vi "Project 11 - MHJ.vi"() -> ()   [LabVIEW 2019]
uses:
  Control 1.ctl
  <vilib>/Waveform/WDTOps.llb/WDT Number of Waveform Samples DBL.vi
  <vilib>/Waveform/WDTOps.llb/WDT Get Waveform Subset DBL.vi
panel:
  out "# Keypad":T1
  in  "Mode":bool
  out "Waveform Chart":dynamicdata(graph)
  in  "stop":bool
  in  "Waveform":waveform(dbl)
  in  "Load File":bool
  out "String":string
  out "Collected Signals":dynamicdata(graph)
  # "RAW SIGNAL"
  # "COLLECTED SIGNAL"
  # "LOAD"
  # "RAW"
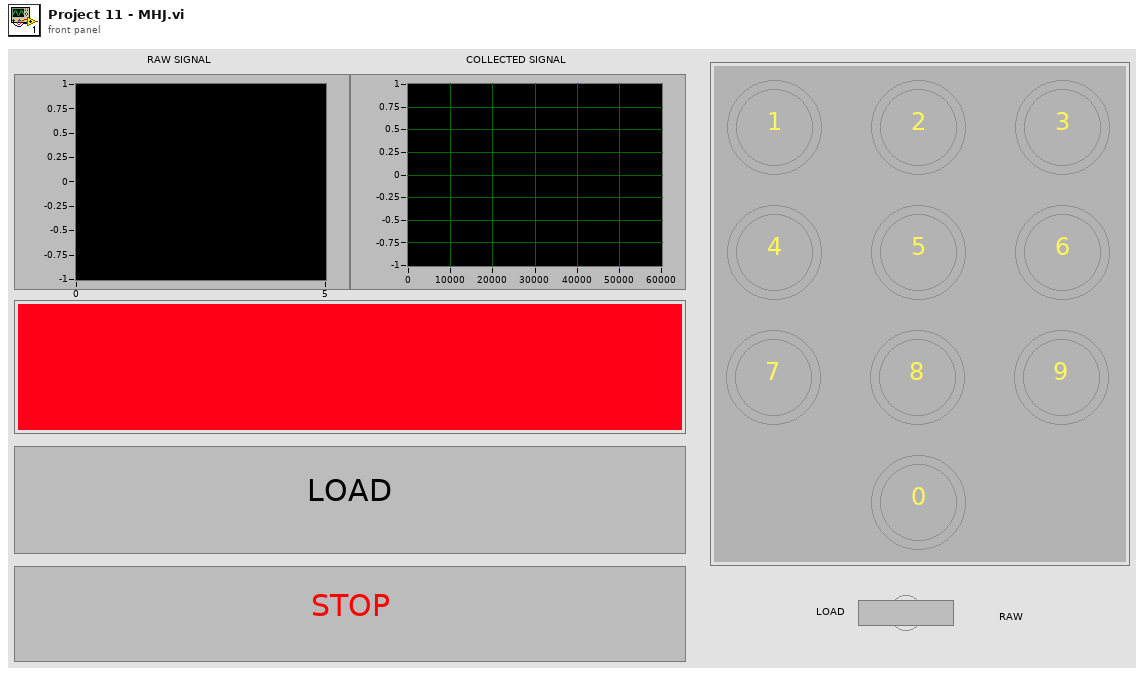
[diagram p1: front panel]
types:
  T1 = cluster{"Boolean 0":bool, "Boolean 9":bool, "Boolean 8":bool, "Boolean 7":bool, "Boolean 6":bool, "Boolean 5":bool, "Boolean 4":bool, "Boolean 3":bool, "Boolean 2":bool, "Boolean 1":bool}
  T2 = typedef "Control 1.ctl" = enum16{"Idle", "Load Image", "Process"}
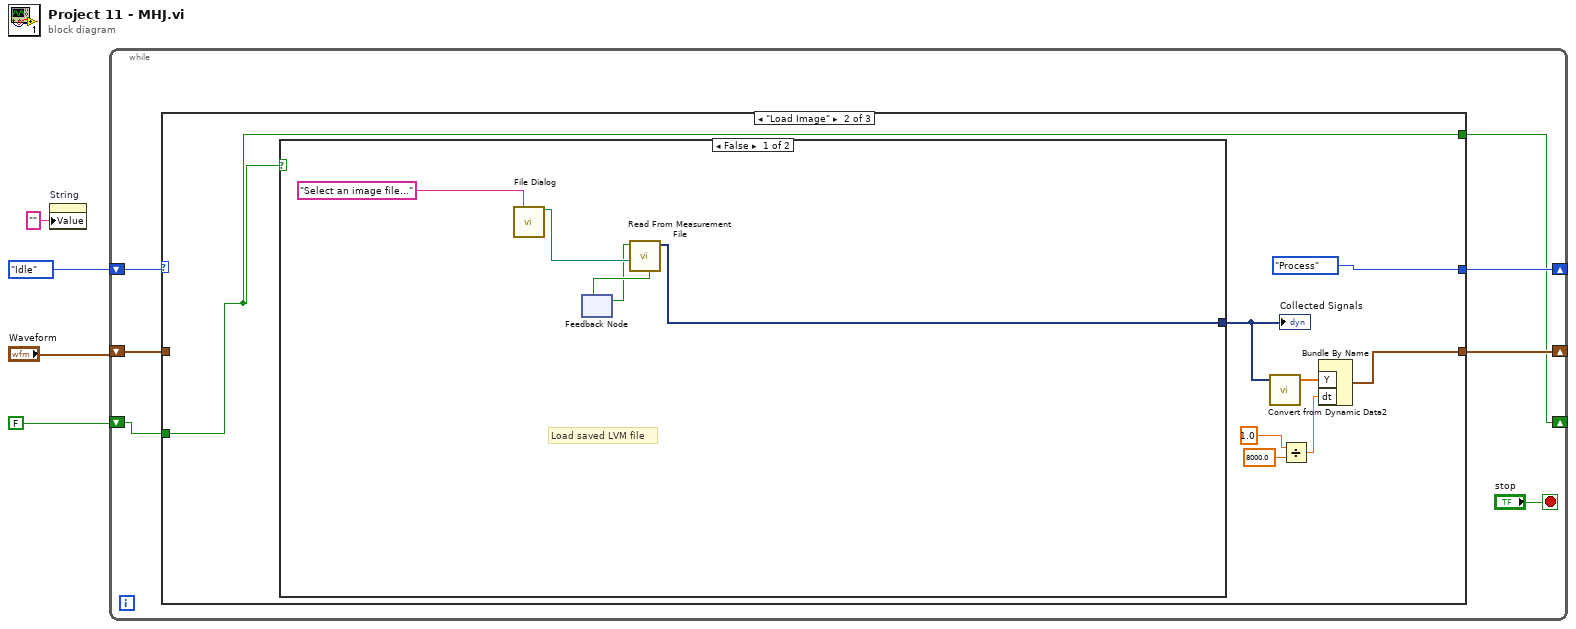
[diagram p0: block diagram]
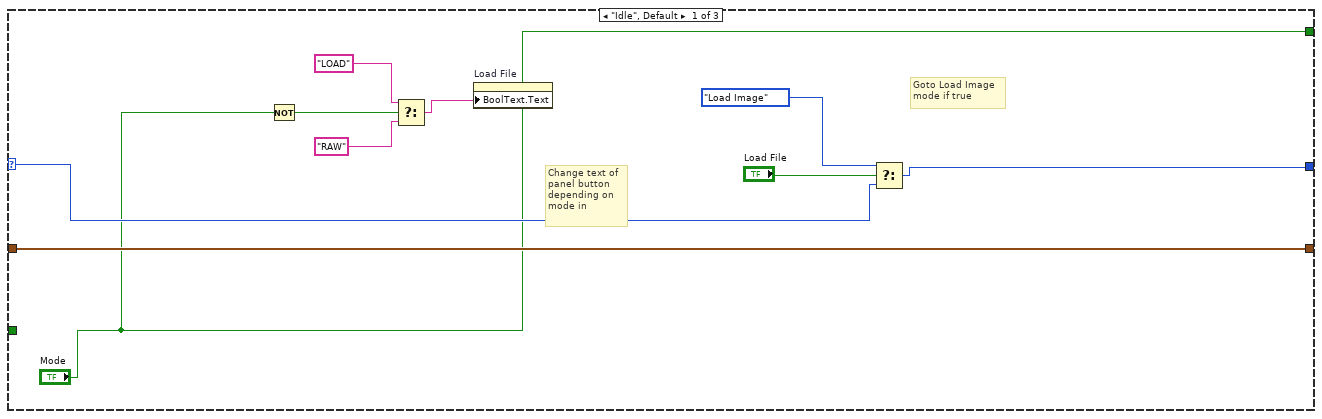
[diagram p2: hidden frame]
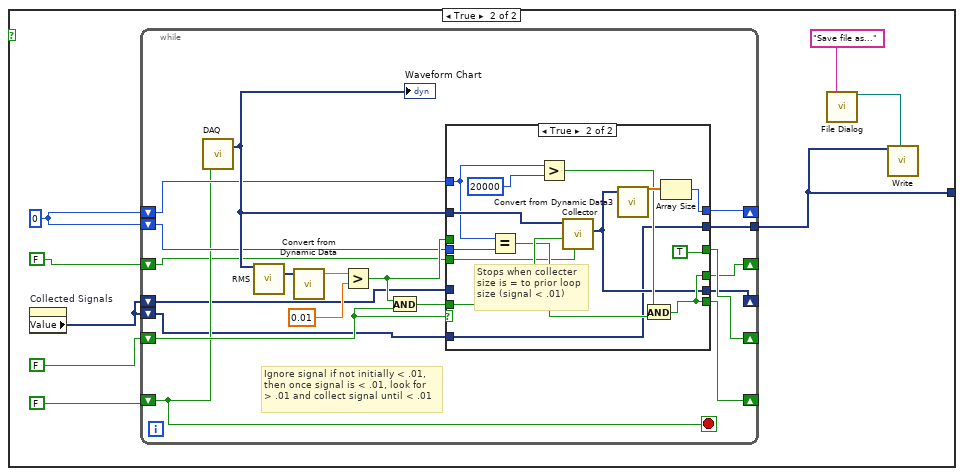
[diagram p3: hidden frame]
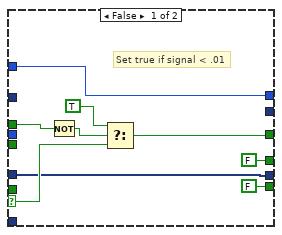
[diagram p4: hidden frame]
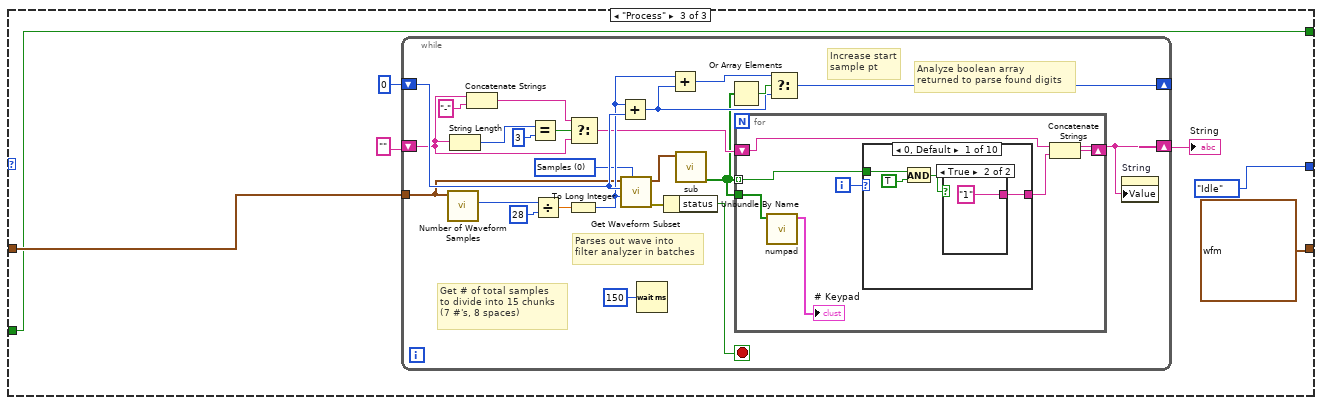
[diagram p5: hidden frame]
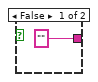
[diagram p6: hidden frame]
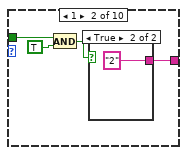
[diagram p7: hidden frame]
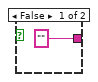
[diagram p8: hidden frame]
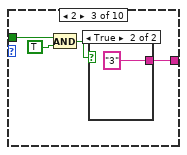
[diagram p9: hidden frame]
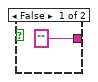
[diagram p10: hidden frame]
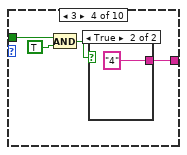
[diagram p11: hidden frame]
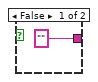
[diagram p12: hidden frame]
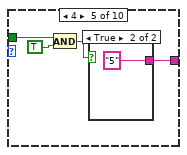
[diagram p13: hidden frame]
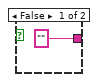
[diagram p14: hidden frame]
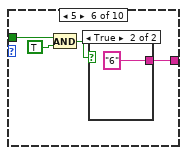
[diagram p15: hidden frame]
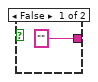
[diagram p16: hidden frame]
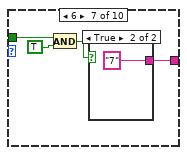
[diagram p17: hidden frame]
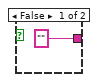
[diagram p18: hidden frame]
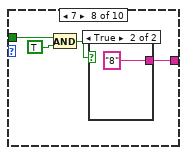
[diagram p19: hidden frame]
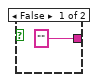
[diagram p20: hidden frame]
diagram:
  n1 = property on="String" class="Str"("Value"="" ("String")) -> ()  [unwired: 2 in, 2 out]
  n2 = while {
    shift-right: [w10] -> _
    shift-left: Control_1."Idle" -> [w11]
    shift-right: [w8] -> _
    shift-left: "Waveform" -> [w9]
    shift-right: [w5] -> _
    shift-left: FALSE -> [w6]
    stop <- "stop" stop-if-true
    n3 = case shown="\"Load Image\"" w11 {
      selector: w11 -> [w20 _ _]
      tunnel: [w18 Control_1."Process" Control_1."Idle"] -> w10
      tunnel: w9 -> [w17 _ w88]
      tunnel: [w17 w22 waveform(dbl) {"t0"=timestamp(0 s since 1904-01-01), "dt"=1.0, "Y"=[]} ("Waveform")] -> w8
      tunnel: w6 -> [_ w28 w85]
      tunnel: ["Mode" w28 w85] -> w5
      frame "Idle", Default {
        # "Goto Load Image\nmode if true"
        # "Change text of\npanel button\ndepending on\nmode in"
        n4 = Not(x="Mode") -> (.not. x?=w12:bool)
        n5 = Select(t="LOAD", s=w12, f="RAW") -> (s? t:f=w16:string)
        n6 = property on="Load File" class="Bool"("BoolText.Text"=w16) -> ()  [unwired: 2 in, 2 out]
        n7 = Select(t=Control_1."Load Image", s="Load File", f=w20) -> (s? t:f=w18:T2)
      }
      frame "Load Image" {
        n8 = case shown="False" w28 {
          tunnel: [w32 w37] -> w23
          frame False {
            # "Load saved LVM file"
            n9 = call "File Dialog"("prompt"="Select an image file...") -> ("selected path"=w33:path)  [unwired: 6 in, 8 out]
            n10 = feedback #1() -> (w30:bool)  [unwired: 1 in]
            n11 = call "Read From Measurement File"("Filename"=w33, "Reset"=w30) -> ("Signals"=w32:dynamicdata, "EOF?"=w31:bool)  [unwired: 4 in, 4 out]
            n12 = feedback-in #1(w31) -> ()
          }
          frame True {
            w41 = 0
            n13 = property on="Collected Signals" class="WFGraph (strict)"() -> ("Value"=w38:dynamicdata)  [unwired: 2 in, 2 out]
            n14 = while {
              tunnel: [w57] -> w37
              shift-right: [w56] -> _
              shift-left: FALSE -> [w54]
              shift-right: [w50] -> _
              shift-left: w41 -> [w52]
              shift-left: w41 -> [w51]
              shift-right: [w43] -> _
              shift-left: FALSE -> [w49]
              shift-right: [w47] -> _
              shift-left: FALSE -> [w48]
              shift-right: [w46] -> _
              shift-left: w38 -> [w44]
              shift-left: w38 -> [w45]
              stop <- w49 stop-if-true
              # "Ignore signal if not initially < .01,\nthen once signal is < .01, look for\n> .01 and collect signal until < .01"
              n15 = call "DAQ"("stop (F)"=w49) -> ("data"=w58:dynamicdata)  [unwired: 15 in, 3 out]
              "Waveform Chart" <- w58
              n16 = call "RMS"("Signals"=w58) -> ("RMS"=w61:dynamicdata)  [unwired: 13 in, 1 out]
              n17 = call "Convert from Dynamic Data"("Dynamic Data Type"=w61) -> ("Scalar"=w59:dbl)  [unwired: 3 in]
              n18 = Greater?(x=w59, y=0.01) -> (0:w55:bool)
              n19 = And(x=w55, y=w54) -> (x .and. y?=w53:bool)
              n20 = case shown="True" w54 {
                selector: w54 -> [w70 _]
                tunnel: w55 -> [w66 _]
                tunnel: w58 -> [_ w84]
                tunnel: [_ w71] -> w57
                tunnel: [w68 TRUE ("t")] -> w56
                tunnel: [FALSE w73] -> w43
                tunnel: w53 -> [_ w82]
                tunnel: w52 -> [w64 w76]
                tunnel: w51 -> [_ w78]
                tunnel: [w64 w75] -> w50
                tunnel: w48 -> [_ w74]
                tunnel: [FALSE w73] -> w47
                tunnel: [w62 w72] -> w46
                tunnel: w45 -> [_ w71]
                tunnel: w44 -> [w62 _]
                frame False {
                  # "Set true if signal < .01"
                  n21 = Not(x=w66) -> (.not. x?=w65:bool)
                  n22 = Select(t=TRUE, s=w65, f=w70) -> (s? t:f=w68:bool)
                }
                frame True {
                  # "Stops when collecter\nsize is = to prior loop\nsize (signal < .01)"
                  n23 = Equal?(x=w76, y=w78) -> (x = y?=w77:bool)
                  n24 = Greater?(x=w76, y=20000) -> (0:w79:bool)
                  n25 = call "Collector"("Reset"=w74, "Enable"=w82, "Signals"=w84) -> ("Collected Signals"=w72:dynamicdata)  [unwired: 7 in, 1 out]
                  n26 = call "Convert from Dynamic Data3"("Dynamic Data Type"=w72) -> ("Array"=w81:dbl[])  [unwired: 3 in]
                  n27 = And(x=w79, y=w77) -> (x .and. y?=w73:bool)
                  n28 = Array Size(array=w81) -> (size(s)=w75:i32)
                }
              }
            }
            n29 = call "File Dialog"("prompt"="Save file as...") -> ("selected path"=w35:path)  [unwired: 6 in, 8 out]
            n30 = call "Write"("Signals"=w37, "Filename"=w35) -> ()  [unwired: 15 in, 3 out]
          }
        }
        "Collected Signals" <- w23
        n31 = call "Convert from Dynamic Data2"("Dynamic Data Type"=w23) -> ("Array"=w27:dbl[])  [unwired: 3 in]
        n32 = Divide(x=1.0, y=8000.0) -> (x/y=w24:dbl)
        n33 = Bundle By Name("Y"=w27, "dt"=w24) -> (w22:waveform(dbl))  [unwired: 1 in]
      }
      frame "Process" {
        n34 = while {
          tunnel: w88 -> [w96]
          shift-right: [w110] -> _
          shift-left: 0 -> [w115]
          shift-right: [w94] -> w91
          shift-left: "" -> [w98]
          stop <- w113 stop-if-true
          w102 = u16 0 items=["Samples", "Relative Time"] ("start/duration format")
          # "Increase start\nsample pt"
          # "Analyze boolean array\nreturned to parse found digits"
          # "Parses out wave into\nfilter analyzer in batches"
          # "Get # of total samples\nto divide into 15 chunks\n(7 #'s, 8 spaces)"
          n35 = call-poly <vilib>:"Number of Waveform Samples.vi"("waveform in"=w96) -> ("number of samples"=w95:i32)  [unwired: 8 in, 2 out]
          n36 = String Length(string=w98) -> (length=w104:i32)
          n37 = Concatenate Strings(w98, "-" ("string")) -> (w99:string)
          n38 = Equal?(x=w104, y=3) -> (x = y?=w101:bool)
          n39 = Divide(x=w95, y=28) -> (x/y=w106:dbl)
          n40 = To Long Integer(number=w106) -> (32bit integer=w105:i32)
          n41 = Select(t=w99, s=w101, f=w98) -> (s? t:f=w100:string)
          n42 = Add(x=w105, y=w115) -> (x+y=w109:i32)
          n43 = call-poly <vilib>:"Get Waveform Subset.vi"("start/duration format"=w102, "duration"=w105, "start samples/time"=w115, "waveform in"=w96) -> ("error out"=w114:errorcluster, "waveform out"=w112:waveform(dbl))  [unwired: 2 in, 2 out]
          n44 = Wait (ms)(milliseconds to wait=u32 150) -> ()  [unwired: 1 out]
          n45 = Unbundle By Name(w114) -> ("status"=w113:bool)
          n46 = Add(x=w105, y=w109) -> (x+y=w108:i32)
          n47 = call "sub.vi"("Waveform Graph 8"=w112) -> ("appended array"=w92:bool[])  [unwired: 9 in, 1 out]
          n48 = Or Array Elements(Boolean array=w92) -> (logical OR=w111:bool)
          n49 = for {
            tunnel: w92 -> [w121] mode=indexing
            shift-right: [w118] -> w94
            shift-left: w100 -> [w120]
            tunnel: w92 -> [w117]
            i -> [w122]
            n50 = call "numpad.vi"("Array"=w117) -> ("Cluster"=→"# Keypad":T1)  [unwired: 10 in]
            n51 = case shown="0, Default" w122 {
              tunnel: w121 -> [w126 w132 w138 w144 w150 w156 w162 w168 w174 w180]
              tunnel: [w123 w129 w135 w141 w147 w153 w159 w165 w171 w177] -> w119
              frame 0, Default {
                n52 = And(x=w126, y=TRUE) -> (x .and. y?=w124:bool)
                n53 = case shown="True" w124 {
                  tunnel: ["" "1"] -> w123
                  frame False {
                  }
                  frame True {
                  }
                }
              }
              frame 1 {
                n54 = And(x=w132, y=TRUE) -> (x .and. y?=w130:bool)
                n55 = case shown="True" w130 {
                  tunnel: ["" "2"] -> w129
                  frame False {
                  }
                  frame True {
                  }
                }
              }
              frame 2 {
                n56 = And(x=w138, y=TRUE) -> (x .and. y?=w136:bool)
                n57 = case shown="True" w136 {
                  tunnel: ["" "3"] -> w135
                  frame False {
                  }
                  frame True {
                  }
                }
              }
              frame 3 {
                n58 = And(x=w144, y=TRUE) -> (x .and. y?=w142:bool)
                n59 = case shown="True" w142 {
                  tunnel: ["" "4"] -> w141
                  frame False {
                  }
                  frame True {
                  }
                }
              }
              frame 4 {
                n60 = And(x=w150, y=TRUE) -> (x .and. y?=w148:bool)
                n61 = case shown="True" w148 {
                  tunnel: ["" "5"] -> w147
                  frame False {
                  }
                  frame True {
                  }
                }
              }
              frame 5 {
                n62 = And(x=w156, y=TRUE) -> (x .and. y?=w154:bool)
                n63 = case shown="True" w154 {
                  tunnel: ["" "6"] -> w153
                  frame False {
                  }
                  frame True {
                  }
                }
              }
              frame 6 {
                n64 = And(x=w162, y=TRUE) -> (x .and. y?=w160:bool)
                n65 = case shown="True" w160 {
                  tunnel: ["" "7"] -> w159
                  frame False {
                  }
                  frame True {
                  }
                }
              }
              frame 7 {
                n66 = And(x=w168, y=TRUE) -> (x .and. y?=w166:bool)
                n67 = case shown="True" w166 {
                  tunnel: ["" "8"] -> w165
                  frame False {
                  }
                  frame True {
                  }
                }
              }
              frame 8 {
                n68 = And(x=w174, y=TRUE) -> (x .and. y?=w172:bool)
                n69 = case shown="True" w172 {
                  tunnel: ["" "9"] -> w171
                  frame False {
                  }
                  frame True {
                  }
                }
              }
              frame 9 {
                n70 = And(x=w180, y=TRUE) -> (x .and. y?=w178:bool)
                n71 = case shown="True" w178 {
                  tunnel: ["" "0"] -> w177
                  frame False {
                  }
                  frame True {
                  }
                }
              }
            }
            n72 = Concatenate Strings(w120, w119) -> (w118:string)
          }
          n73 = Select(t=w108, s=w111, f=w109) -> (s? t:f=w110:i32)
          n74 = property on="String" class="Str"("Value"=w94) -> ()  [unwired: 2 in, 2 out]
        }
        "String" <- w91
      }
    }
  }
